vi "Update Input.vi"(8 "error in (no error)":errorcluster, 10 "Input Control":T1, 11 "CallVIStep in":refnum<class "CallVIStep.lvclass">) -> (0 "error out":errorcluster, 3 "CallVIStep out":refnum<class "CallVIStep.lvclass">)   [LabVIEW 2015, in "CallVIStep.lvclass"]
uses:
  CallVIStep.lvclass
  VI Input Control Typedef.ctl
  VI Input Type Typedef.ctl
  VI Input Typedef.ctl
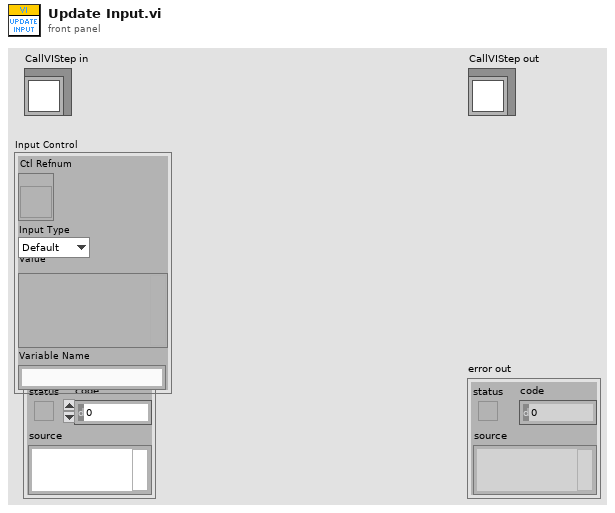
[diagram p1: front panel]
types:
  T1 = typedef "CallVIStep.lvclass/VI Input Control Typedef.ctl" = cluster{"Ctl Refnum":refnum<vi>, "Input Type":T2, "Value":variant, "Variable Name":string}
  T2 = typedef "CallVIStep.lvclass/VI Input Type Typedef.ctl" = enum16{"Default", "Value", "Variable"}
  T3 = typedef "CallVIStep.lvclass/VI Input Typedef.ctl" = cluster{"Label":string, "Input Type":T2, "Type String":i16[], "Data String":string, "Variable Name":string}
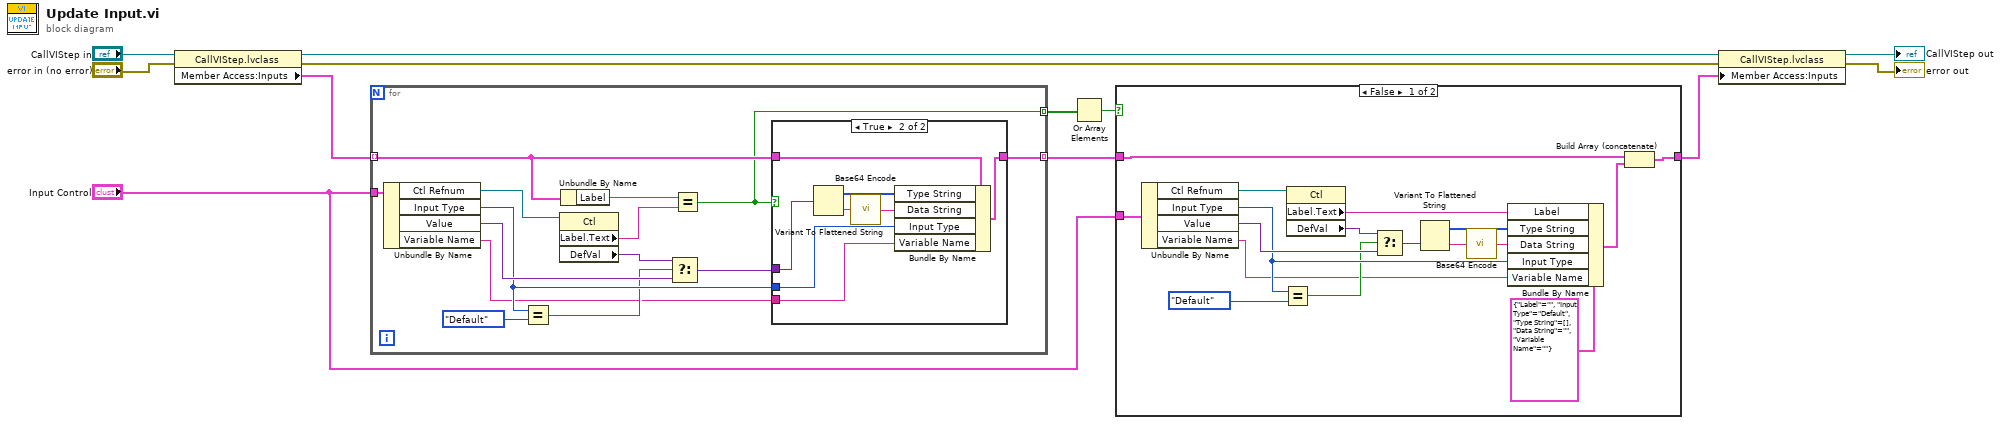
[diagram p0: block diagram]
diagram:
  n1 = property class="CallVIStep.lvclass"(reference="CallVIStep in", error in="error in (no error)") -> (reference out=w3:refnum<class "CallVIStep.lvclass">, error out=w2:errorcluster, "Member Access:Inputs"=w1:T3[])
  n2 = for {
    tunnel: w1 -> [w22] mode=indexing
    tunnel: "Input Control" -> [w26]
    tunnel: [w19] -> w10 mode=indexing
    tunnel: [w17] -> w12 mode=indexing
    n3 = Unbundle By Name(w26) -> ("Ctl Refnum"=w25:refnum<vi>, "Input Type"=w16:T2, "Value"=w21:variant, "Variable Name"=w13:string)
    n4 = Equal?(x=w16, y=VI_Input_Type_Typedef."Default") -> (x = y?=w14:bool)
    n5 = property class="Ctl"(reference=w25) -> ("Label.Text"=w23:string, "DefVal"=w18:variant)  [unwired: 1 in, 2 out]
    n6 = Unbundle By Name(w22) -> ("Label"=w24:string)
    n7 = Select(t=w18, s=w14, f=w21) -> (s? t:f=w20:variant)
    n8 = Equal?(x=w24, y=w23) -> (x = y?=w17:bool)
    n9 = case shown="True" w17 {
      tunnel: w22 -> [w27 w35]
      tunnel: w20 -> [_ w32]
      tunnel: w16 -> [_ w34]
      tunnel: [w27 w33] -> w19
      tunnel: w13 -> [_ w28]
      frame False {
      }
      frame True {
        n10 = Variant To Flattened String(Variant=w32) -> (data string=w30:string, 1:w31:i16[])
        n11 = call "Base64 Encode.vi"("normal string"=w30) -> ("base64 string"=w29:string)  [unwired: 1 in]
        n12 = Bundle By Name(cluster=w35, "Type String"=w31, "Data String"=w29, "Input Type"=w34, "Variable Name"=w28) -> (w33:T3)
      }
    }
  }
  n13 = Or Array Elements(Boolean array=w12) -> (logical OR=w11:bool)
  n14 = case shown="False" w11 {
    tunnel: w10 -> [w52 w53]
    tunnel: [w51 w53] -> w8
    tunnel: "Input Control" -> [w49 _]
    frame False {
      n15 = Unbundle By Name(w49) -> ("Ctl Refnum"=w48:refnum<vi>, "Input Type"=w39:T2, "Value"=w45:variant, "Variable Name"=w36:string)
      n16 = Equal?(x=w39, y=VI_Input_Type_Typedef."Default") -> (x = y?=w38:bool)
      n17 = property class="Ctl"(reference=w48) -> ("Label.Text"=w47:string, "DefVal"=w46:variant)  [unwired: 1 in, 2 out]
      n18 = Select(t=w46, s=w38, f=w45) -> (s? t:f=w43:variant)
      n19 = Variant To Flattened String(Variant=w43) -> (data string=w41:string, 1:w42:i16[])
      n20 = call "Base64 Encode.vi"("normal string"=w41) -> ("base64 string"=w40:string)  [unwired: 1 in]
      n21 = Bundle By Name(cluster=T3 {"Label"="", "Input Type"=enum."Default", "Type String"=[], "Data String"="", "Variable Name"=""} ("Input"), "Label"=w47, "Type String"=w42, "Data String"=w40, "Input Type"=w39, "Variable Name"=w36) -> (w50:T3)
      n22 = Build Array (concatenate)(w52, w50) -> (w51:T3[])
    }
    frame True {
    }
  }
  n23 = property class="CallVIStep.lvclass"(reference=w3, error in=w2, "Member Access:Inputs"=w8) -> (reference out=→"CallVIStep out":refnum<class "CallVIStep.lvclass">, error out=→"error out":errorcluster)
